vi "ProcessDataFlow.vi"(7 "Qbus in":refnum<class "Qbus.lvclass">, 8 "error in (no error)":errorcluster, 10 "Data":T6, 11 "config in":T1={"DataSet Type"=enum."Waveform", "ChanNameMap"=variant, "Common"={"State"=enum."On", "Waveform Channel"="", "DataGroup"="", "Number of Samples"=0, "Waveform Length (sec)"=0.0, "Timeout"=0.0, "History"=variant, "LastRequest"=timestamp(0 s since 1904-01-01), "BufferSize"=0, "OpState"=variant, "IRoutingSource"={"CorrelationId"="", "ReplyTo"=""}}}) -> (0 "error out":errorcluster, 3 "config out":T1={"DataSet Type"=enum."Waveform", "ChanNameMap"=variant, "Common"={"State"=enum."On", "Waveform Channel"="", "DataGroup"="", "Number of Samples"=0, "Waveform Length (sec)"=0.0, "Timeout"=0.0, "History"=variant, "LastRequest"=timestamp(0 s since 1904-01-01), "BufferSize"=0, "OpState"=variant, "IRoutingSource"={"CorrelationId"="", "ReplyTo"=""}}})   [LabVIEW 2017, in "EmsaTestPanel.lvlib"]
uses:
  <vilib>/addons/InsightCM/Devices/Shared/Emsa/EmsaTestPanel/EmsaTestPanel.lvlib
  <vilib>/addons/InsightCM/Devices/Shared/Emsa/EmsaTestPanel/controls/Configuration.ctl
  <vilib>/addons/InsightCM/Devices/Shared/Emsa/EmsaTestPanel/controls/DataSetType.ctl
  <vilib>/addons/InsightCM/Devices/Shared/Common/TestPanel/controls/Configuration.ctl
  <vilib>/addons/InsightCM/Devices/Shared/Common/TestPanel/controls/State.ctl
  <vilib>/addons/InsightCM/MessageBus/Base/controls/IRoutingSource.ctl
  <vilib>/addons/InsightCM/Devices/Shared/Common/DataFlow/controls/Data.ctl
  <vilib>/addons/InsightCM/Utilities/DataAccessors/controls/wfmSGL_DVR.ctl
  <vilib>/addons/PointValueMap/controls/PointMap.ctl
  <vilib>/addons/InsightCM/Devices/Shared/Common/DataFlow/controls/Type.ctl
  <vilib>/addons/Qbus/Qbus.lvclass
  <vilib>/addons/InsightCM/MessageBus/MessageLibrary/Device/controls/DeviceTestPanelGetDataSetForChannelResponseBody.ctl
  <vilib>/addons/InsightCM/MessageBus/Base/controls/DataSetByteData.ctl
  <vilib>/addons/InsightCM/MessageBus/Base/controls/KeyValuePair.ctl
  <vilib>/addons/InsightCM/Devices/Shared/Common/ServerComm/ServerComm.lvlib
  <vilib>/addons/InsightCM/Devices/Shared/Common/TestPanel/TestPanel.lvlib
  <vilib>/addons/InsightCM/Devices/Shared/Common/DataFlow/DataFlow.lvlib
  <vilib>/addons/PointValueMap/PointValueMap.lvlib
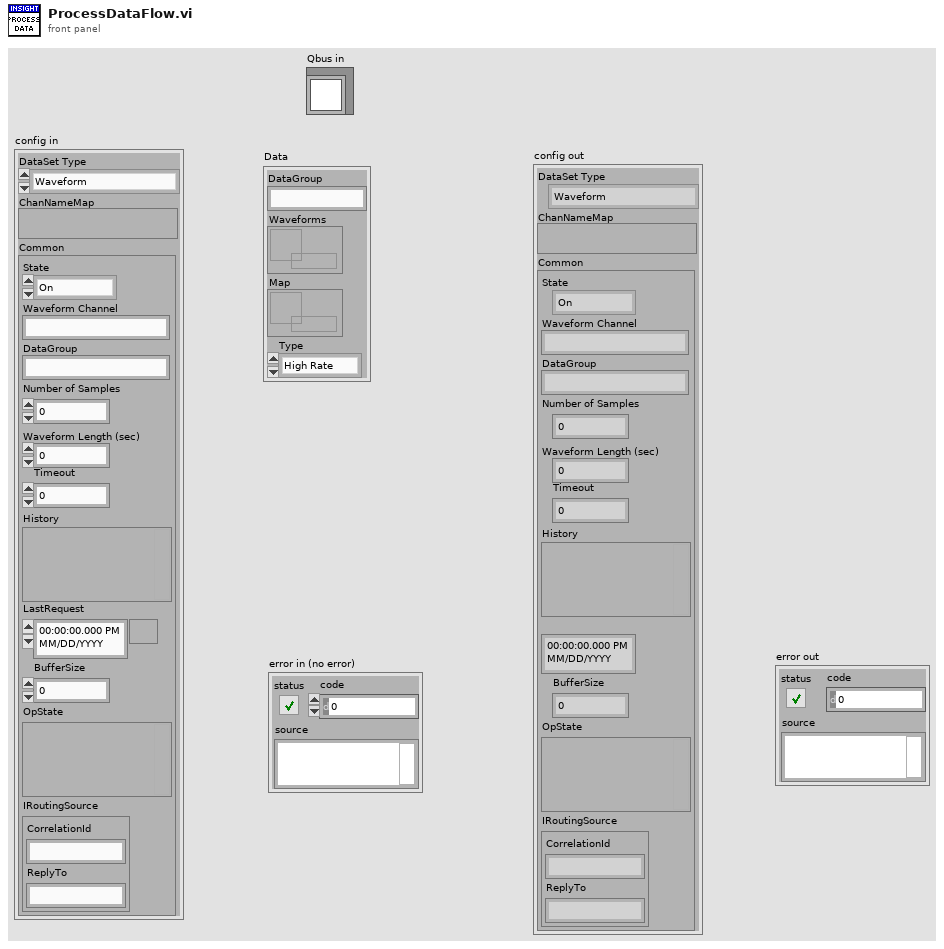
[diagram p1: front panel]
types:
  T1 = typedef "EmsaTestPanel.lvlib/Configuration.ctl" = cluster{"DataSet Type":T2, "ChanNameMap":variant, "Common":T3}
  T2 = typedef "EmsaTestPanel.lvlib/DataSetType.ctl" = enum16{"Waveform", "Sweep", "WAV"}
  T3 = typedef "TestPanel.lvlib/Configuration.ctl" = cluster{"State":T4, "Waveform Channel":string, "DataGroup":string, "Number of Samples":i32, "Waveform Length (sec)":dbl, "Timeout":dbl, "History":variant, "LastRequest":timestamp, "BufferSize":i32, "OpState":variant, "IRoutingSource":T5}
  T4 = typedef "TestPanel.lvlib/State.ctl" = enum16{"Off", "On", "PendingValues", "PendingDataSet"}
  T5 = typedef "IRoutingSource.ctl" = cluster{"CorrelationId":string, "ReplyTo":string}
  T6 = typedef "DataFlow.lvlib/Data.ctl" = cluster{"DataGroup":string, "Waveforms":T7, "Map":T8, "Type":T9}
  T7 = typedef "wfmSGL_DVR.ctl" = refnum<data-value>
  T8 = typedef "PointValueMap.lvlib/PointMap.ctl" = refnum<data-value>
  T9 = typedef "DataFlow.lvlib/Type.ctl" = enum16{"High Rate", "Low Rate", "Burst Mode"}
  T10 = typedef "DeviceTestPanelGetDataSetForChannelResponseBody.ctl" = cluster{"DataSet":T11}
  T11 = typedef "DataSetByteData.ctl" = cluster{"Id":string, "DataEventId":string, "AssetNodeId":string, "Type":string, "T0":i64, "Props":T12[], "DataBase64":string}
  T12 = typedef "KeyValuePair.ctl" = cluster{"Key":string, "Value":string}
  T13 = typedef "Message.ctl" = cluster{"Header":T14, "Body":u8[]}
  T14 = typedef "MessageHeader.ctl" = cluster{"MessageName":string, "Timestamp":i64, "CorrelationId":string, "ContentType":string, "RoutingKey":string, "Properties":T12[]}
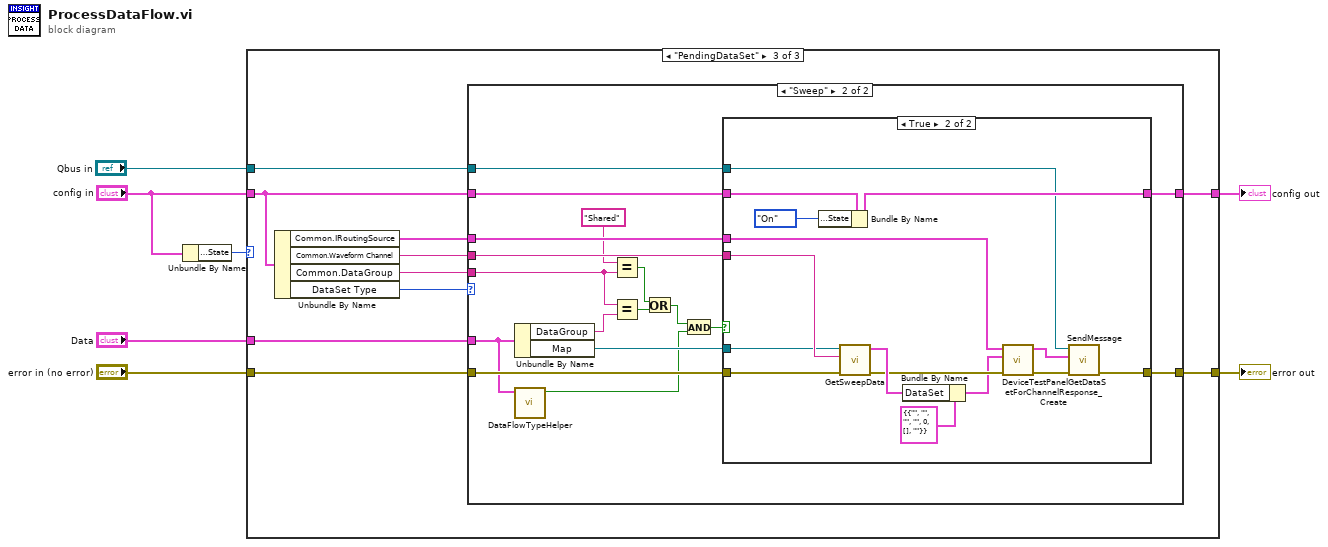
[diagram p0: block diagram]
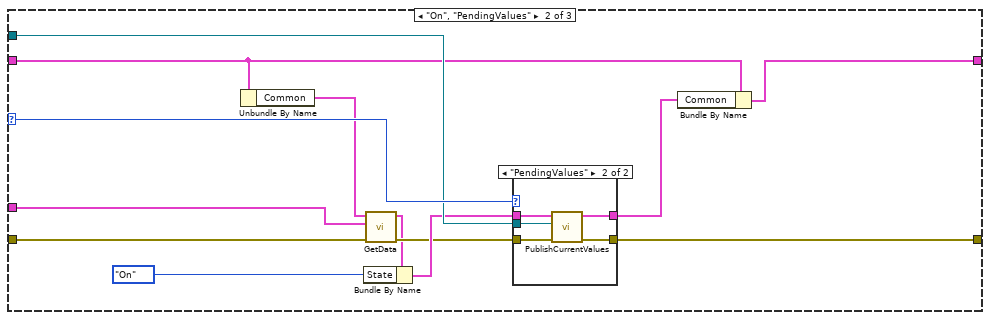
[diagram p3: hidden frame]
diagram:
  n1 = Unbundle By Name("config in") -> ("Common.State"=w7:T4)
  n2 = case shown="\"PendingDataSet\"" w7 {
    selector: w7 -> [_ w22 _]
    tunnel: "error in (no error)" -> [w8 w18 w39]
    tunnel: [w8 w21 w33] -> w2
    tunnel: "config in" -> [w9 w12 w36]
    tunnel: "Data" -> [_ w17 w37]
    tunnel: [w9 w10 w35] -> w3
    tunnel: "Qbus in" -> [_ w20 w34]
    frame "Off" {
    }
    frame "On", "PendingValues" {
      n3 = Unbundle By Name(w12) -> ("Common"=w16:T3)
      n4 = call <vilib>:"GetData.vi"("error in (no error)"=w18, "Data"=w17, "config in"=w16) -> ("error out"=w15:errorcluster, "config out"=w14:T3)  [unwired: 7 in]
      n5 = Bundle By Name(cluster=w14, "State"=State."On" ("Test Panel State")) -> (w19:T3)
      n6 = case shown="\"PendingValues\"" w22 {
        tunnel: w19 -> [w23 w27]
        tunnel: w15 -> [w24 w29]
        tunnel: [w24 w28] -> w21
        tunnel: [w23 w25] -> w11
        tunnel: w20 -> [_ w26]
        frame Default {
        }
        frame "PendingValues" {
          n7 = call <vilib>:"PublishCurrentValues.vi"("error in (no error)"=w29, "Qbus in"=w26, "config in"=w27) -> ("error out"=w28:errorcluster, "config out"=w25:T3)  [unwired: 7 in]
        }
      }
      n8 = Bundle By Name(cluster=w12, "Common"=w11) -> (w10:T1)
    }
    frame "PendingDataSet" {
      n9 = Unbundle By Name(w36) -> ("Common.IRoutingSource"=w32:T5, "Common.Waveform Channel"=w38:string, "Common.DataGroup"=w31:string, "DataSet Type"=w30:T2)
      n10 = case shown="\"Sweep\"" w30 {
        tunnel: w39 -> [w40 w58]
        tunnel: w38 -> [_ w57]
        tunnel: w37 -> [_ w43]
        tunnel: w36 -> [w41 w56]
        tunnel: [w41 w55] -> w35
        tunnel: w34 -> [_ w54]
        tunnel: [w40 w53] -> w33
        tunnel: w32 -> [_ w52]
        tunnel: w31 -> [_ w49]
        frame Default {
        }
        frame "Sweep" {
          n11 = Unbundle By Name(w43) -> ("DataGroup"=w51:string, "Map"=w44:T8)
          n12 = call <vilib>:"DataFlowTypeHelper.vi"("data"=w43) -> ("high rate"=w42:bool)  [unwired: 8 in, 2 out]
          n13 = Equal?(x="Shared", y=w49) -> (x = y?=w48:bool)
          n14 = Equal?(x=w49, y=w51) -> (x = y?=w50:bool)
          n15 = Or(x=w48, y=w50) -> (x .or. y?=w46:bool)
          n16 = And(x=w46, y=w42) -> (x .and. y?=w45:bool)
          n17 = case shown="True" w45 {
            tunnel: w58 -> [w60 w75]
            tunnel: w57 -> [_ w74]
            tunnel: w56 -> [w59 w73]
            tunnel: [w59 w72] -> w55
            tunnel: w54 -> [_ w71]
            tunnel: [w60 w66] -> w53
            tunnel: w52 -> [_ w64]
            tunnel: w44 -> [_ w61]
            frame False {
            }
            frame True {
              n18 = Bundle By Name(cluster=w73, "Common.State"=State."On" ("Test Panel State")) -> (w72:T1)
              n19 = call <vilib>:"GetSweepData.vi"("error in (no error)"=w75, "Current Channel"=w74, "map"=w61) -> ("error out"=w67:errorcluster, "DataSet"=w69:T11)  [unwired: 7 in]
              n20 = Bundle By Name(cluster=T10 {"DataSet"={"Id"="", "DataEventId"="", "AssetNodeId"="", "Type"="", "T0"=0, "Props"=[], "DataBase64"=""}} ("DeviceTestPanelGetWaveformChannelResponse"), "DataSet"=w69) -> (w65:T10)
              n21 = call <vilib>:"DeviceTestPanelGetDataSetForChannelResponse_Create.vi"("error in (no error)"=w67, "DeviceTestPanelGetDataSetForChannelResponse"=w65, "IRoutingSource"=w64) -> ("error out"=w68:errorcluster, "Message"=w63:T13)  [unwired: 7 in]
              n22 = call <vilib>:"SendMessage.vi"("error in (no error)"=w68, "message"=w63, "Qbus in"=w71) -> ("error out"=w66:errorcluster)  [unwired: 7 in, 1 out]
            }
          }
        }
      }
    }
  }
  "error out" <- w2
  "config out" <- w3
